vi "niDTS BT INSTR TX UTIL Average Type ModAcc.vi"(7 "Average In":T1(ring)) -> (8 "Average Out":enum16{"RMS", "MAX", "MIN"}(ring))   [LabVIEW 2015, in "niDTS BT.lvlib" / "niDTS BT INSTR TX.lvclass"]
uses:
  niDTS BT INSTR TX.lvclass
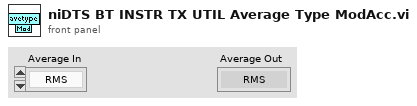
[diagram p1: front panel]
types:
  T1 = enum16{"RMS", "LOG", "SCALAR", "MAX", "MIN", "VECTOR"}
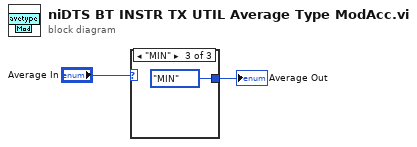
[diagram p0: block diagram]
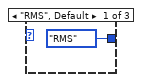
[diagram p2: hidden frame]
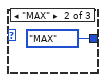
[diagram p3: hidden frame]
diagram:
  n1 = case shown="\"MIN\"" "Average In" {
    tunnel: [enum16{"RMS", "MAX", "MIN"}."RMS" ("Average Out") enum16{"RMS", "MAX", "MIN"}."MAX" ("Average Out") enum16{"RMS", "MAX", "MIN"}."MIN" ("Average Out")] -> w1
    frame "RMS", Default {
    }
    frame "MAX" {
    }
    frame "MIN" {
    }
  }
  "Average Out" <- w1
